vi "ParseRobotMoves.vi"(11 "file path (dialog if empty)":path) -> (2 "Array":T1(array[cluster]))   [LabVIEW 2012]
uses:
  <vilib>/Utility/file.llb/Read From Spreadsheet File (string).vi
panel:
  in  "Cluster":T2 {"Y Joystick Value" scale=1.0..-1.0; "X Joystick Value" scale=-1.0..1.0}
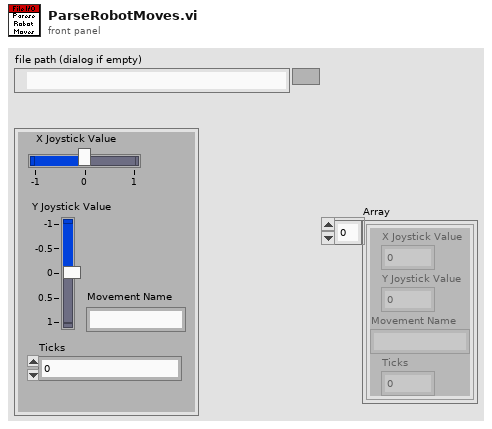
[diagram p1: front panel]
types:
  T1 = cluster{"X Joystick Value":dbl, "Y Joystick Value":dbl, "Movement Name":string, "Ticks":dbl}[]
  T2 = cluster{"X Joystick Value":dbl, "Y Joystick Value":dbl, "Movement Name":string, "Ticks":dbl}
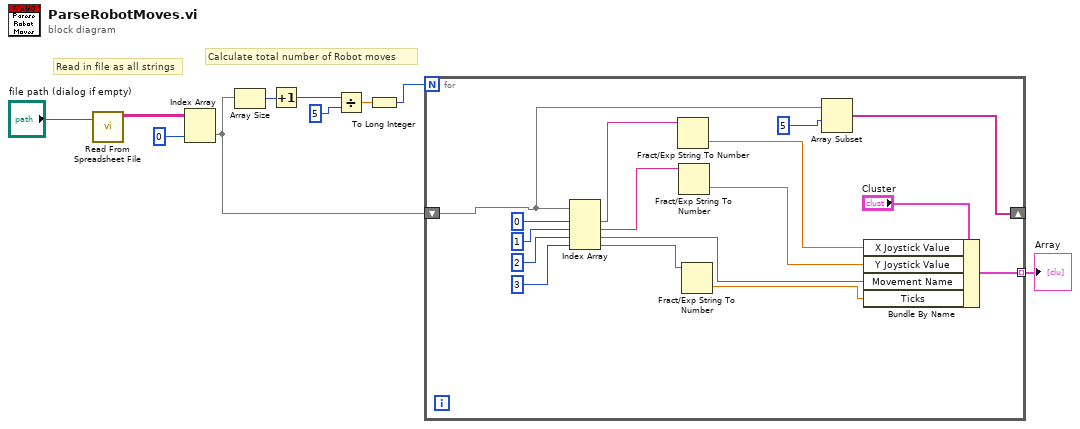
[diagram p0: block diagram]
diagram:
  # "Calculate total number of Robot moves"
  # "Read in file as all strings"
  n1 = call-poly <vilib>:"Read From Spreadsheet File.vi"("file path (dialog if empty)"="file path (dialog if empty)") -> ("all rows"=w9:string[][])  [unwired: 6 in, 4 out]
  n2 = Index Array(array=w9, index (col)=0 ("disabled index (col)")) -> (element=w2:string[])  [unwired: 1 in]
  n3 = Array Size(array=w2) -> (size(s)=w6:i32)
  n4 = Increment(x=w6) -> (x+1=w5:i32)
  n5 = Divide(x=w5, y=5) -> (x/y=w3:dbl)
  n6 = To Long Integer(number=w3) -> (32bit integer=w4:i32)
  n7 = for {
    N: w4 -> [_]
    tunnel: [w18] -> w1 mode=indexing
    shift-right: [w16] -> _
    shift-left: w2 -> [w17]
    n8 = Index Array(array=w17, index #1=0 ("index"), index #2=1 ("index"), index #3=2 ("index"), index #4=3 ("index")) -> (element #1=w21:string, element #2=w22:string, element #3=w12:string, element #4=w13:string)
    n9 = Fract/Exp String To Number(string=w21) -> (number=w20:dbl)  [unwired: 3 in, 1 out]
    n10 = Fract/Exp String To Number(string=w22) -> (number=w19:dbl)  [unwired: 3 in, 1 out]
    n11 = Fract/Exp String To Number(string=w13) -> (number=w11:dbl)  [unwired: 3 in, 1 out]
    n12 = Array Subset(array=w17, index=5 ("length")) -> (w16:string[])  [unwired: 1 in]
    n13 = Bundle By Name(cluster="Cluster", "X Joystick Value"=w20, "Y Joystick Value"=w19, "Movement Name"=w12, "Ticks"=w11) -> (w18:T2)
  }
  "Array" <- w1
